vi "unConstrainedNonLinearOptimizationForChi2.vi"(3 "output control":T2, 4 "data":T4, 5 "X":dbl[](array[numeric])) -> (0 "error out":errorcluster, 1 "gradient":dbl[](array[numeric]), 2 "f(X)":dbl)   [LabVIEW 2013]
doc: "This template is the starting point for creating an objective function, equality constraint function and inequality constraint function to be passed to the Constrained Nonlinear Optimization.vi."
uses:
  <vilib>/gmath/NumericalOptimization/objective function data.ctl
  BaesDataTypeDefinition.ctl
  <vilib>/gmath/NI_Gmath.lvlib
panel:
  out "Enum":T1(ring)
  in  "Extinction ExtinctionUncertainity Size parameter and Number ofS sizes 2":T3={"Extinction"=[], "Extinction Uncertainty"=[], "Size parameters"=[], "Number ofSizes"=0.0, "GeometricCrossSection"=[], "Wave Length"=0.0, "SMPS Sizes"=[], "Concentration"=[], "Double Charge Correction"=FALSE, "Extincation Factor"=1.0, "Diameter Factor"=1.0, "Diameter Offset"=0.0, "Extinction Factor Flag"=FALSE, "Diameter Factor Flag"=FALSE, "Diameter Offset Flag"=FALSE, "Sizes"=[], "ExtinctionOrAbsorptionOrScattering"=0, "Convergence Strength"=enum."Weak"} {"ExtinctionOrAbsorptionOrScattering" scale=0.0..2.0}
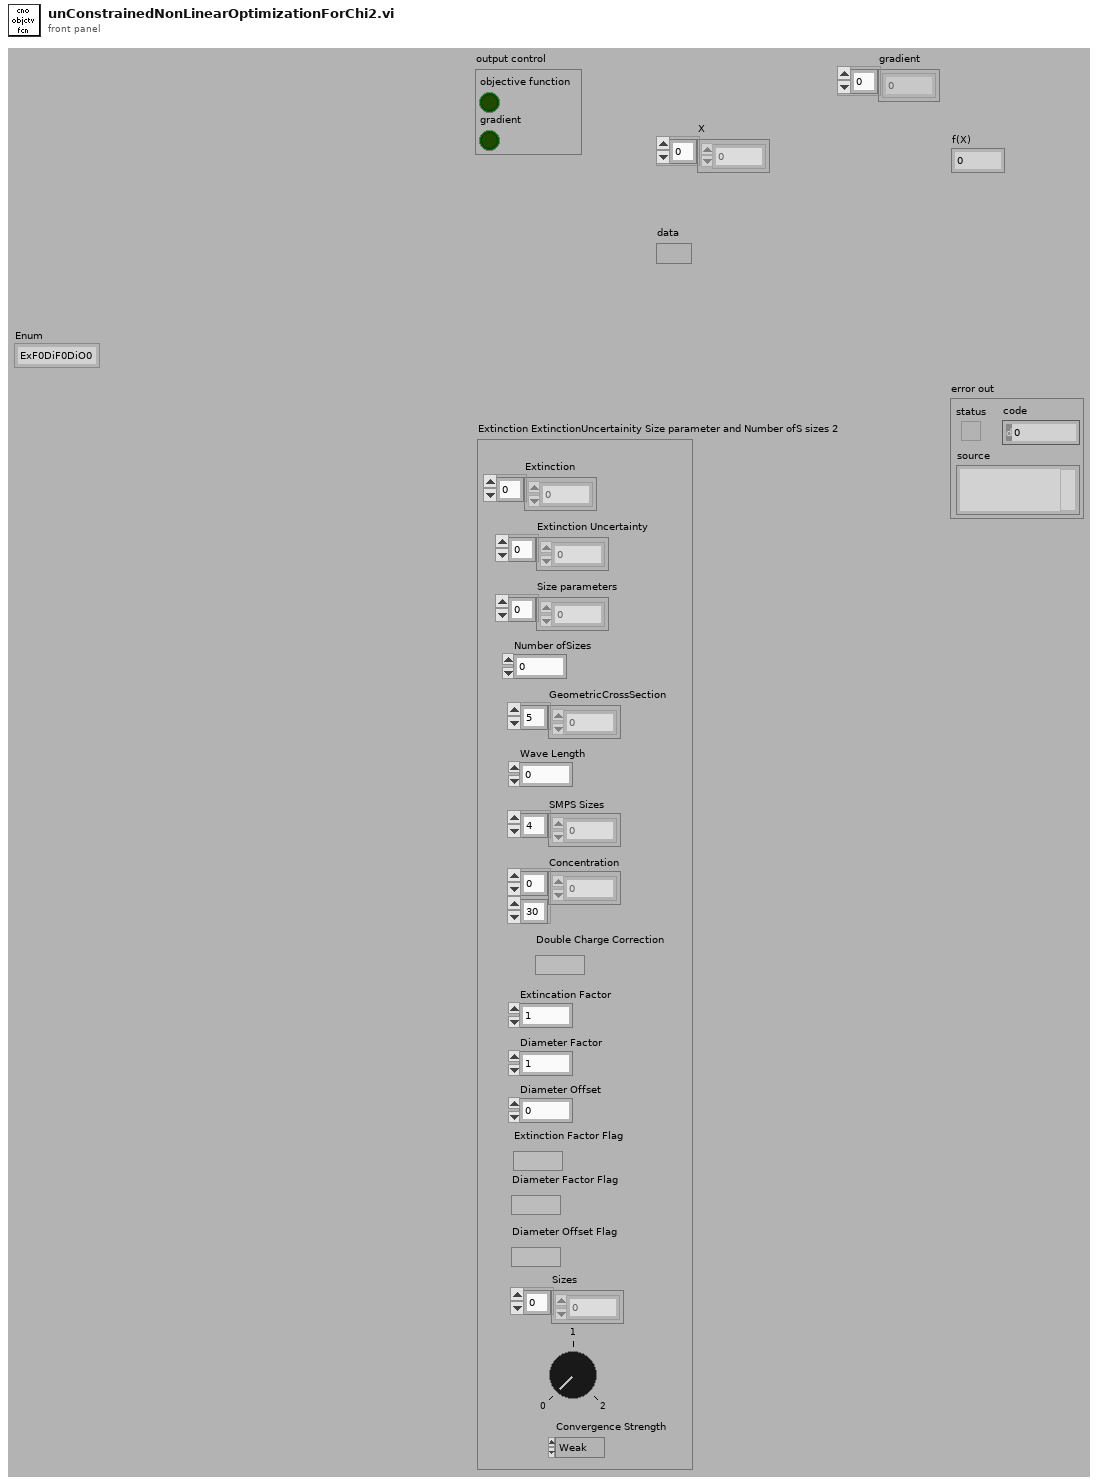
[diagram p1: front panel]
types:
  T1 = enum16{"ExF0DiF0DiO0", "ExF0DiF0DiO1", "ExF0DiF1DiO0", "NotDefined1", "ExF1DiF0DiO0", "ExF1DiF0DiO1", "ExF1DiF1DiO0", "NotDefined"}
  T2 = cluster{"objective function":bool, "gradient":bool}
  T3 = typedef "BaesDataTypeDefinition.ctl" = cluster{"Extinction":dbl[], "Extinction Uncertainty":dbl[], "Size parameters":dbl[], "Number ofSizes":dbl, "GeometricCrossSection":dbl[], "Wave Length":dbl, "SMPS Sizes":dbl[], "Concentration":dbl[][], "Double Charge Correction":bool, "Extincation Factor":dbl, "Diameter Factor":dbl, "Diameter Offset":dbl, "Extinction Factor Flag":bool, "Diameter Factor Flag":bool, "Diameter Offset Flag":bool, "Sizes":dbl[], "ExtinctionOrAbsorptionOrScattering":i8, "Convergence Strength":enum16{"Weak", "Medium", "Strong"}}
  T4 = typedef "NI_Gmath.lvlib/objective function data.ctl" = variant
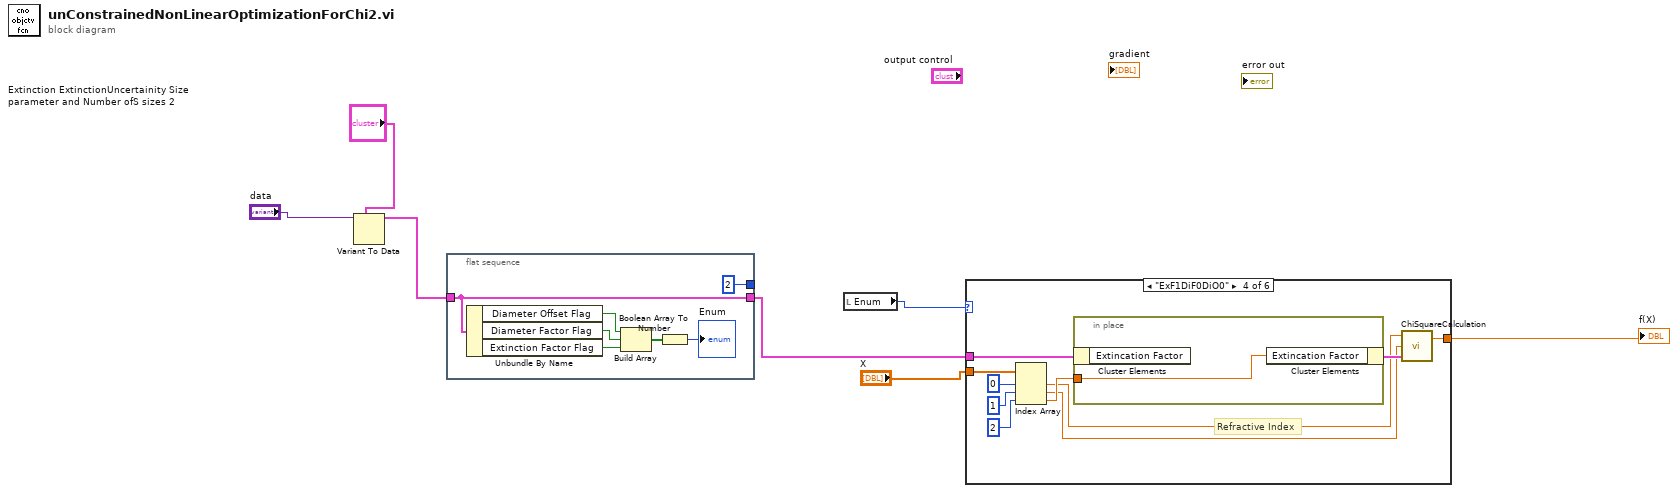
[diagram p0: block diagram]
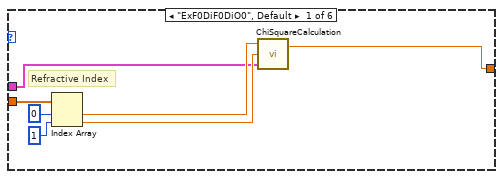
[diagram p2: hidden frame]
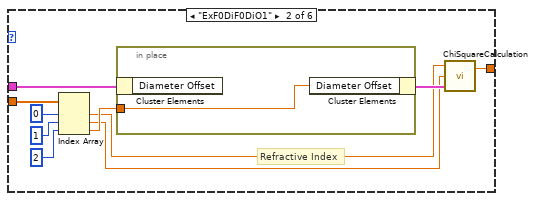
[diagram p3: hidden frame]
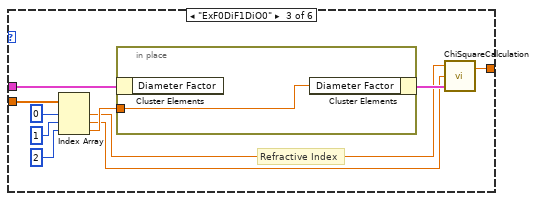
[diagram p4: hidden frame]
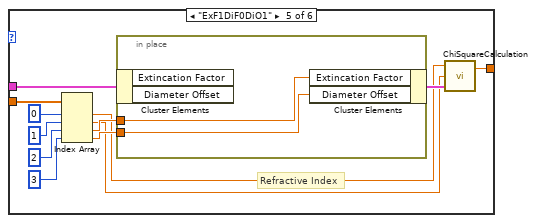
[diagram p5: hidden frame]
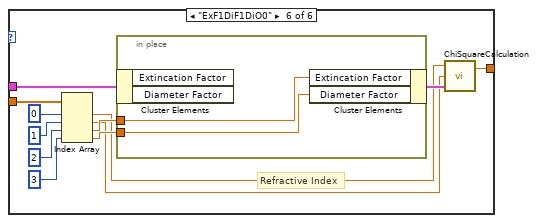
[diagram p6: hidden frame]
diagram:
  n1 = Variant To Data(type="Extinction ExtinctionUncertainity Size parameter and Number ofS sizes 2", Variant="data") -> (data=w5:T3)  [unwired: 1 in, 1 out]
  n2 = flat-sequence {
    tunnel: [2 ("index")] -> _
    tunnel: w5 -> [w8]
    tunnel: [w8] -> w3
    frame #0 {
      n3 = Unbundle By Name(w8) -> ("Diameter Offset Flag"=w13:bool, "Diameter Factor Flag"=w12:bool, "Extinction Factor Flag"=w11:bool)
      n4 = Build Array(w13, w12, w11) -> (w10:bool[])
      n5 = Boolean Array To Number(Boolean array=w10) -> (number=→"Enum":u32)
    }
  }
  n6 = local read "Enum"() -> (w2:T1)
  n7 = case shown="\"ExF1DiF0DiO0\"" w2 {
    tunnel: w3 -> [w16 w29 w38 w49 w62 w74]
    tunnel: [w15 w22 w33 w44 w55 w69] -> w1
    tunnel: "X" -> [w19 w26 w37 w48 w59 w73]
    frame "ExF0DiF0DiO0", Default {
      # "Refractive Index"
      n8 = Index Array(array=w19, index #1=0 ("index"), index #2=1 ("index")) -> (element #1=w18:dbl, element #2=w17:dbl)
      n9 = call "ChiSquareCalculation.vi"("Extinction ExtinctionUncertainity Size parameter and Number ofS sizes 2"=w16, "refractive index, imaginary"=w17, "refractive index, real"=w18) -> ("Chi Squared"=w15:dbl)  [unwired: 1 out]
    }
    frame "ExF0DiF0DiO1" {
      # "Refractive Index"
      n10 = Index Array(array=w26, index #1=0 ("index"), index #2=1 ("index"), index #3=2 ("index")) -> (element #1=w24:dbl, element #2=w23:dbl, element #3=w27:dbl)
      n11 = in-place {
        in-place-border: w27 -> [w32]
        n12 = in-place-cluster #1(w29) -> ()  [unwired: 1 out]
        n13 = in-place-cluster #1("Diameter Offset"=w32) -> (w25:T3)
      }
      n14 = call "ChiSquareCalculation.vi"("Extinction ExtinctionUncertainity Size parameter and Number ofS sizes 2"=w25, "refractive index, imaginary"=w23, "refractive index, real"=w24) -> ("Chi Squared"=w22:dbl)  [unwired: 1 out]
    }
    frame "ExF0DiF1DiO0" {
      # "Refractive Index"
      n15 = Index Array(array=w37, index #1=0 ("index"), index #2=1 ("index"), index #3=2 ("index")) -> (element #1=w35:dbl, element #2=w34:dbl, element #3=w39:dbl)
      n16 = in-place {
        in-place-border: w39 -> [w43]
        n17 = in-place-cluster #2(w38) -> ()  [unwired: 1 out]
        n18 = in-place-cluster #2("Diameter Factor"=w43) -> (w36:T3)
      }
      n19 = call "ChiSquareCalculation.vi"("Extinction ExtinctionUncertainity Size parameter and Number ofS sizes 2"=w36, "refractive index, imaginary"=w34, "refractive index, real"=w35) -> ("Chi Squared"=w33:dbl)  [unwired: 1 out]
    }
    frame "ExF1DiF0DiO0" {
      # "Refractive Index"
      n20 = Index Array(array=w48, index #1=0 ("index"), index #2=1 ("index"), index #3=2 ("index")) -> (element #1=w46:dbl, element #2=w45:dbl, element #3=w50:dbl)
      n21 = in-place {
        in-place-border: w50 -> [w54]
        n22 = in-place-cluster #3(w49) -> ()  [unwired: 1 out]
        n23 = in-place-cluster #3("Extincation Factor"=w54) -> (w47:T3)
      }
      n24 = call "ChiSquareCalculation.vi"("Extinction ExtinctionUncertainity Size parameter and Number ofS sizes 2"=w47, "refractive index, imaginary"=w45, "refractive index, real"=w46) -> ("Chi Squared"=w44:dbl)  [unwired: 1 out]
    }
    frame "ExF1DiF0DiO1" {
      # "Refractive Index"
      n25 = Index Array(array=w59, index #1=0 ("index"), index #2=1 ("index"), index #3=2 ("index"), index #4=3 ("index")) -> (element #1=w57:dbl, element #2=w56:dbl, element #3=w63:dbl, element #4=w60:dbl)
      n26 = in-place {
        in-place-border: w63 -> [w68]
        in-place-border: w60 -> [w67]
        n27 = in-place-cluster #4(w62) -> ()  [unwired: 2 out]
        n28 = in-place-cluster #4("Extincation Factor"=w68, "Diameter Offset"=w67) -> (w58:T3)
      }
      n29 = call "ChiSquareCalculation.vi"("Extinction ExtinctionUncertainity Size parameter and Number ofS sizes 2"=w58, "refractive index, imaginary"=w56, "refractive index, real"=w57) -> ("Chi Squared"=w55:dbl)  [unwired: 1 out]
    }
    frame "ExF1DiF1DiO0" {
      # "Refractive Index"
      n30 = Index Array(array=w73, index #1=0 ("index"), index #2=1 ("index"), index #3=2 ("index"), index #4=3 ("index")) -> (element #1=w71:dbl, element #2=w70:dbl, element #3=w77:dbl, element #4=w75:dbl)
      n31 = in-place {
        in-place-border: w77 -> [w82]
        in-place-border: w75 -> [w81]
        n32 = in-place-cluster #5(w74) -> ()  [unwired: 2 out]
        n33 = in-place-cluster #5("Extincation Factor"=w82, "Diameter Factor"=w81) -> (w72:T3)
      }
      n34 = call "ChiSquareCalculation.vi"("Extinction ExtinctionUncertainity Size parameter and Number ofS sizes 2"=w72, "refractive index, imaginary"=w70, "refractive index, real"=w71) -> ("Chi Squared"=w69:dbl)  [unwired: 1 out]
    }
  }
  "f(X)" <- w1
